vi "EventClient_RaiseEvent.vi"(6 "Top Priority":bool, 8 "error in (no error)":errorcluster, 10 "Data":variant, 11 "Event":string) -> (0 "error out":errorcluster)   [LabVIEW 2018]
uses:
  EventClient_ObjectReference.ctl
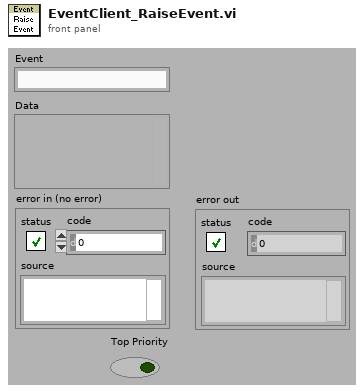
[diagram p1: front panel]
types:
  T1 = typedef "EventClient_ObjectReference.ctl" = refnum<k1>
  T2 = cluster{"Client":refnum<queue>, "Sub Events":string[], "PrvData":variant, "MyName":string}
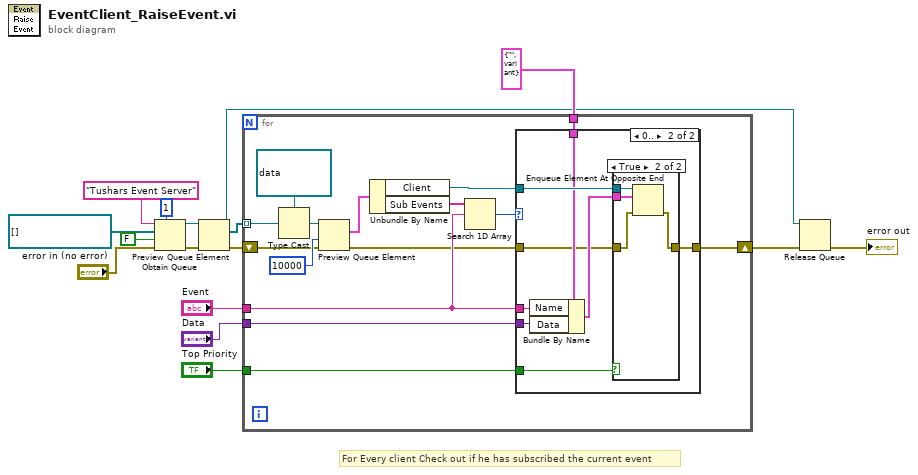
[diagram p0: block diagram]
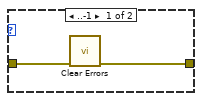
[diagram p2: hidden frame]
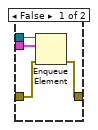
[diagram p3: hidden frame]
diagram:
  w12 = T1[] [] items=["EventClient"]
  # "For Every client Check out if he has subscribed the current event"
  n1 = Obtain Queue(max queue size (-1, unlimited)=1, name (unnamed)="Tushars Event Server", element data type=w12, create if not found? (T)=FALSE, error in (no error)="error in (no error)") -> (queue out=w14:refnum<queue>, error out=w15:errorcluster)  [unwired: 1 out]
  n2 = Preview Queue Element(queue=w14, error in (no error)=w15) -> (queue out=w1:refnum<queue>, element=w11:T1[], error out=w10:errorcluster)  [unwired: 2 out]
  n3 = for {
    tunnel: w11 -> [w31] mode=indexing
    shift-right: [w19] -> w3
    shift-left: w10 -> [w27]
    tunnel: "Event" -> [w21]
    tunnel: cluster{"Name":string, "Data":variant} {"Name"="", "Data"=variant} ("element") -> [w22]
    tunnel: "Data" -> [w20]
    tunnel: "Top Priority" -> [w17]
    n4 = Type Cast(type=refnum<queue> refnum ("queue out"), x=w31) -> (*(type *) &x=w30:refnum<queue>)
    n5 = Preview Queue Element(queue=w30, timeout in ms (-1)=10000, error in (no error)=w27) -> (element=w29:T2, error out=w18:errorcluster)  [unwired: 2 out]
    n6 = Unbundle By Name(w29) -> ("Client"=w23:refnum<queue>, "Sub Events"=w25:string[])
    n7 = Search 1D Array(1D array=w25, element=w21) -> (index of element=w24:i32)  [unwired: 1 out]
    n8 = case shown="0.." w24 {
      tunnel: w23 -> [_ w41]
      tunnel: w22 -> [_ w40]
      tunnel: w21 -> [_ w39]
      tunnel: w20 -> [_ w38]
      tunnel: [w32 w35] -> w19
      tunnel: w18 -> [w33 w36]
      tunnel: w17 -> [_ w34]
      frame ..-1 {
        n9 = call <vilib>:"Clear Errors.vi"("error in (no error)"=w33) -> ("error out"=w32:errorcluster)  [unwired: 1 in, 5 out]
      }
      frame 0.. {
        n10 = Bundle By Name(cluster=w40, "Name"=w39, "Data"=w38) -> (w37:cluster{"Name":string, "Data":variant})
        n11 = case shown="True" w34 {
          tunnel: w41 -> [w45 w49]
          tunnel: w37 -> [w44 w48]
          tunnel: w36 -> [w43 w47]
          tunnel: [w42 w46] -> w35
          frame False {
            n12 = Enqueue Element(queue=w45, element=w44, error in (no error)=w43) -> (error out=w42:errorcluster)  [unwired: 3 out]
          }
          frame True {
            n13 = Enqueue Element At Opposite End(queue=w49, element=w48, error in (no error)=w47) -> (error out=w46:errorcluster)  [unwired: 3 out]
          }
        }
      }
    }
  }
  n14 = Release Queue(queue=w1, error in (no error)=w3) -> (error out=→"error out":errorcluster)  [unwired: 3 out]
